vi "Min_get.vi"(9 "Current Min":dbl, 10 "on/off":bool, 11 "Current Value":dbl) -> (2 "new min ping":bool, 3 "New Min":dbl)   [LabVIEW 2019]
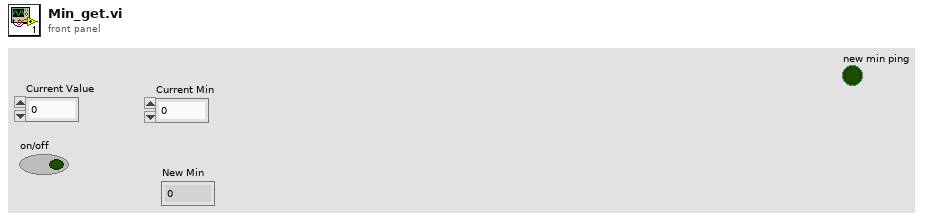
[diagram p1: front panel]
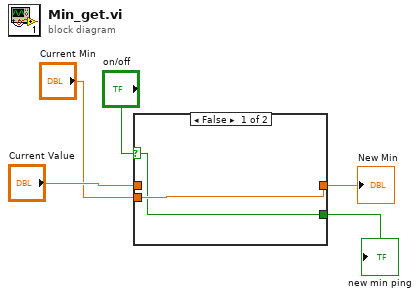
[diagram p0: block diagram]
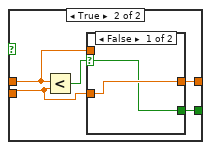
[diagram p2: hidden frame]
diagram:
  n1 = case shown="False" "on/off" {
    selector: "on/off" -> [w6 _]
    tunnel: "Current Value" -> [_ w11]
    tunnel: "Current Min" -> [w7 w10]
    tunnel: [w7 w9] -> w2
    tunnel: [w6 w8] -> w1
    frame False {
    }
    frame True {
      n2 = Less?(x=w11, y=w10) -> (x < y?=w12:bool)
      n3 = case shown="False" w12 {
        selector: w12 -> [w13 w15]
        tunnel: w11 -> [_ w16]
        tunnel: w10 -> [w14 _]
        tunnel: [w14 w16] -> w9
        tunnel: [w13 w15] -> w8
        frame False {
        }
        frame True {
        }
      }
    }
  }
  "New Min" <- w2
  "new min ping" <- w1
